vi "Actor Core.vi"(8 "error in":errorcluster, 11 "Splitter Settings UI in":refnum<class "Splitter Settings UI.lvclass">) -> (0 "error out":errorcluster, 3 "Actor out":refnum<class "Actor.lvclass">)   [LabVIEW 2020, in "Splitter Settings UI.lvlib" / "Splitter Settings UI.lvclass"]
doc: "The user interface for this panel.\n\n----\nPlease see the following web address for additional documentation and tutorial information:\nhttp://www.mooregoodideas.com/mgi-panel-manager/\n\nAuthor: Derek Trepanier\n\nCopyright (c) 2018, Moore Good Ideas, Inc.\n\nAll rights reserved.\n\nRedistribution and use in source and binary forms, with or without modification, are permitted provided that the following conditions are met:\n\n * Redistributions of source code must retain the above copyright notice, this list of conditions and the following disclaimer.\n * Redistributions in binary form must reproduce the above copyright notice, this list of conditions and the following disclaimer in the documentation and/or other materials provided with the distribution.\n * Neither the name of Moore Good Ideas, Inc. nor the names of its contributors may be used to endorse or promote products derived from this software without specific prior written permission.\n\nTHIS SOFTWARE IS PROVIDED BY THE COPYRIGHT HOLDERS AND CONTRIBUTORS \"AS IS\" AND ANY EXPRESS OR IMPLIED WARRANTIES, INCLUDING, BUT NOT LIMITED TO, THE IMPLIED WARRANTIES OF MERCHANTABILITY AND FITNESS FOR A PARTICULAR PURPOSE ARE DISCLAIMED. IN NO EVENT SHALL THE COPYRIGHT OWNER OR CONTRIBUTORS BE LIABLE FOR ANY DIRECT, INDIRECT, INCIDENTAL, SPECIAL, EXEMPLARY, OR CONSEQUENTIAL DAMAGES (INCLUDING, BUT NOT LIMITED TO, PROCUREMENT OF SUBSTITUTE GOODS OR SERVICES; LOSS OF USE, DATA, OR PROFITS; OR BUSINESS INTERRUPTION) HOWEVER CAUSED AND ON ANY THEORY OF LIABILITY, WHETHER IN CONTRACT, STRICT LIABILITY, OR TORT (INCLUDING NEGLIGENCE OR OTHERWISE) ARISING IN ANY WAY OUT OF THE USE OF THIS SOFTWARE, EVEN IF ADVISED OF THE POSSIBILITY OF SUCH DAMAGE."
uses:
  Splitter Settings UI.lvclass
  C:/Program Files (x86)/National Instruments/LabVIEW 2020/vi.lib/MGI/Panel Manager/Panel Actor/Panel Actor/Panel Actor.lvclass
  C:/Program Files (x86)/National Instruments/LabVIEW 2020/vi.lib/ActorFramework/Actor/Actor.lvclass
  <vilib>/ActorFramework/Actor/Actor.lvclass
  Typedefs/Splitter Style--Enum.ctl
  Splitter/Splitter.lvclass
  <vilib>/ActorFramework/Actor/Actor.lvclass/Actor.ctl
  <vilib>/ActorFramework/Message Enqueuer/Message Enqueuer.lvclass/Message Enqueuer.ctl
  Splitter Settings UI.lvclass/Splitter Settings UI.ctl
  Splitter Settings UI Messages/Set Cursor Busy State Msg/Set Cursor Busy State Msg.lvclass/Set Cursor Busy State Msg.ctl
  <vilib>/ActorFramework/Message Enqueuer/Init from Existing Queue.vi
  <vilib>/ActorFramework/Message Enqueuer/Enqueue.vi
  Pane Relief Main UI/Pane Relief Main UI Messages/Panel Object Settings Changed Msg/Panel Object Settings Changed Msg.lvclass
  C:/Program Files (x86)/National Instruments/LabVIEW 2020/vi.lib/ActorFramework/Message/Message.lvclass
  Splitter Settings UI Messages/Set Cursor Busy State Msg/Set Cursor Busy State Msg.lvclass
  <vilib>/ActorFramework/Message Priority Queue/Priority Enqueue.vi
  <vilib>/ActorFramework/Message Enqueuer/Message Enqueuer.lvclass
  <vilib>/MGI/Panel Manager/Panel Actor/Panel Actor/Panel Actor.lvclass
panel:
  in  "Label":string
  in  "Refresh Style Value":bool
  in  "Style":T1 items=["Modern", "Classic", "System", "NXG"]
  in  "Size":i32 min=0
  in  "Color":u32(colorbox)
  in  "Locked":bool
  in  "Sizing":u16(ring) items=["Sticks Top", "Sticks Bottom", "Proportional"]
  in  "Position":i32
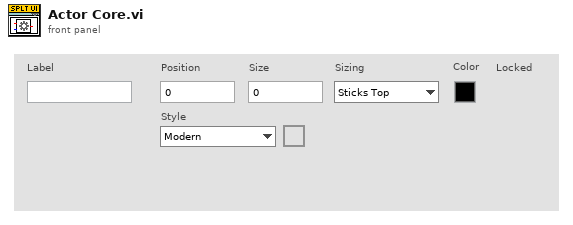
[diagram p1: front panel]
types:
  T1 = typedef "Splitter Style--Enum.ctl" = u16
  T2 = cluster{"Event Registration Refnum":refnum<event-registration>, "Pnl Actor":refnum<event-registration>}
  T3 = typedef "Splitter Sizing--Enum.ctl" = enum16{"Sticks Top/Left", "Sticks Bottom/Right", "Proportional"}
  T4 = typedef "Splitter Orientation--Enum.ctl" = enum16{"Vertical", "Horizontal"}
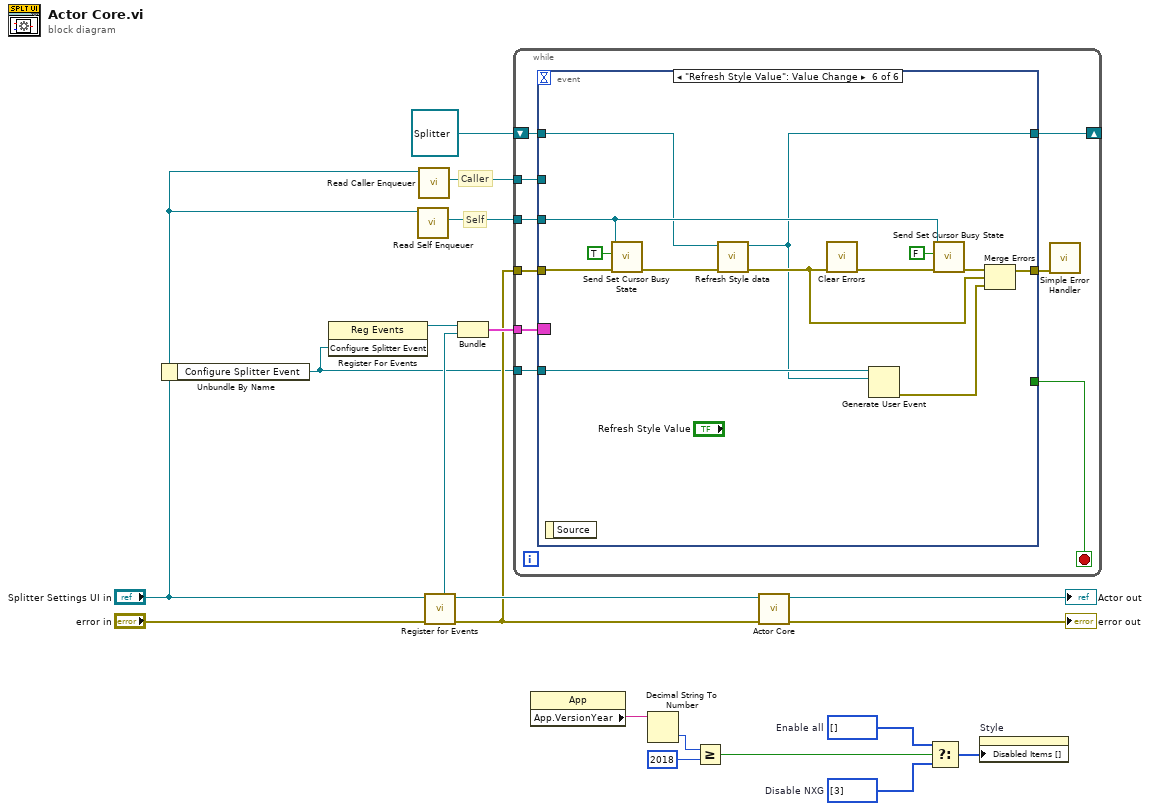
[diagram p0: block diagram]
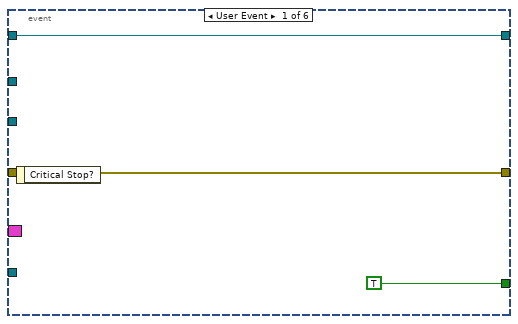
[diagram p2: hidden frame]
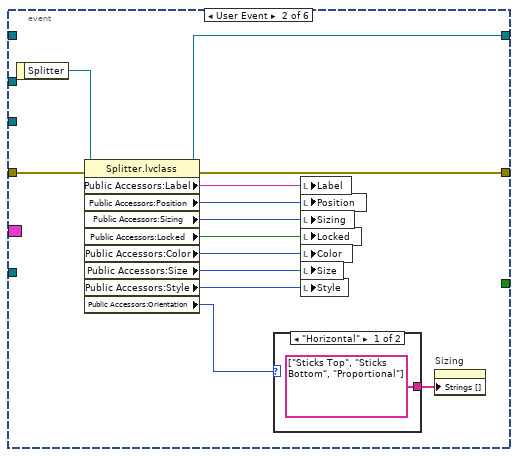
[diagram p3: hidden frame]
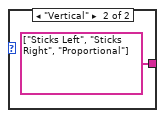
[diagram p4: hidden frame]
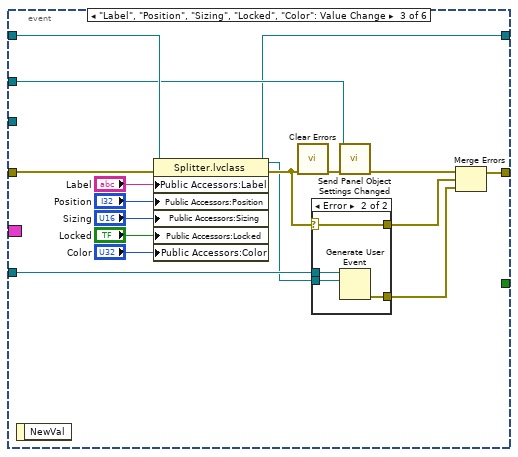
[diagram p5: hidden frame]
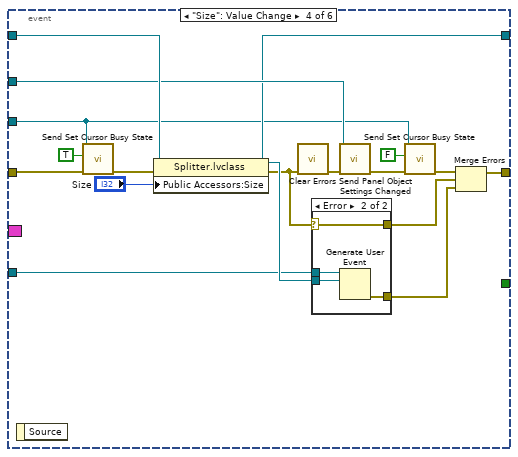
[diagram p7: hidden frame]
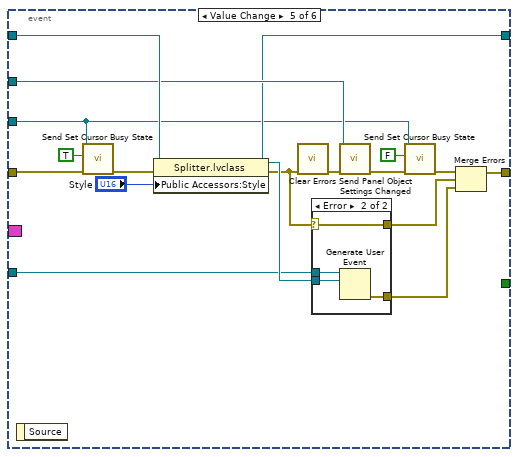
[diagram p9: hidden frame]
diagram:
  w3 = i32[] []  # Enable all
  w2 = i32[] [3]  # Disable NXG
  # "Self"
  # "Caller"
  n1 = Unbundle By Name("Splitter Settings UI in") -> ("Configure Splitter Event"=w10:refnum<user-event>)
  n2 = register-events(w10) -> (reference out=w16:refnum<event-registration>)  [unwired: 2 in, 1 out]
  n3 = call <vilib>:"Read Self Enqueuer.vi"("Actor"="Splitter Settings UI in") -> ("Self Enqueuer"=w9:refnum<class "Message Enqueuer.lvclass">)  [unwired: 10 in]
  n4 = call <vilib>:"Read Caller Enqueuer.vi"("Actor"="Splitter Settings UI in") -> ("Caller Enqueuer"=w11:refnum<class "Message Enqueuer.lvclass">)  [unwired: 10 in]
  n5 = call <vilib>:"Register for Events.vi"("Error In"="error in", "Panel Actor in"="Splitter Settings UI in") -> ("Error Out"=w12:errorcluster, "Panel Actor out"=w18:refnum<class "Splitter Settings UI.lvclass">, "Pnl Actor"=w15:refnum<event-registration>)  [unwired: 6 in, 1 out]
  n6 = Bundle("Event Registration Refnum"=w16, "Pnl Actor"=w15) -> (w14:T2)  [unwired: 1 in]
  n7 = while {
    tunnel: w14 -> [w29]
    shift-right: [w27] -> _
    shift-left: refnum<class "Splitter.lvclass"> refnum ("Splitter.lvclass") -> [w26]
    tunnel: w11 -> [w24]
    tunnel: w12 -> [w25]
    tunnel: w10 -> [w22]
    tunnel: w9 -> [w21]
    stop <- w28 stop-if-true
    n8 = event shown="[5] \"Refresh Style Value\": Value Change" {
      selector: w29 -> [_ _ _ _ _ _]
      dyn-events: _ -> [_ _ _ _ _ _]
      timeout: _ -> [_ _ _ _ _ _]
      tunnel: [TRUE _ _ _ _ _] -> w28
      tunnel: [w32 w38 w49 w78 w101 w113] -> w27
      tunnel: w26 -> [w32 _ w57 w85 w107 w114]
      tunnel: w25 -> [w31 w40 w58 w73 w96 w120]
      tunnel: [w31 w39 w53 w82 w105 w125] -> w23
      tunnel: w24 -> [_ _ w55 w81 w104 _]
      tunnel: w22 -> [_ _ w50 w76 w99 w122]
      tunnel: w21 -> [_ _ _ w71 w94 w118]
      event User Event {
        n9 = event-data() -> ()  [unwired: 1 in, 1 out]
      }
      event User Event {
        n10 = event-data() -> ("Splitter"=w37:refnum<class "Splitter.lvclass">)  [unwired: 1 in]
        n11 = property class="Splitter.lvclass"(reference=w37, error in=w40) -> (reference out=w38:refnum<class "Splitter.lvclass">, error out=w39:errorcluster, "Public Accessors:Label"=w45:string, "Public Accessors:Position"=w44:i32, "Public Accessors:Sizing"=w43:T3, "Public Accessors:Locked"=w42:bool, "Public Accessors:Color"=w41:u32, "Public Accessors:Size"=w36:i32, "Public Accessors:Style"=w33:T1, "Public Accessors:Orientation"=w35:T4)
        n12 = case shown="\"Horizontal\"" w35 {
          tunnel: [string[] ["Sticks Top", "Sticks Bottom", "Proportional"] ("Strings []") string[] ["Sticks Left", "Sticks Right", "Proportional"] ("Strings []")] -> w34
          frame "Horizontal" {
          }
          frame "Vertical" {
          }
        }
        n13 = local write "Label"(w45) -> ()
        n14 = local write "Position"(w44) -> ()
        n15 = local write "Sizing"(w43) -> ()
        n16 = local write "Locked"(w42) -> ()
        n17 = local write "Color"(w41) -> ()
        n18 = local write "Size"(w36) -> ()
        n19 = local write "Style"(w33) -> ()
        n20 = property on="Sizing" class="Ring (strict)"("Strings []"=w34) -> ()  [unwired: 2 in, 2 out]
      }
      event "Label", "Position", "Sizing", "Locked", "Color": Value Change {
        n21 = event-data() -> ()  [unwired: 1 in, 1 out]
        n22 = property class="Splitter.lvclass"(reference=w57, error in=w58, "Public Accessors:Label"="Label", "Public Accessors:Position"="Position", "Public Accessors:Sizing"="Sizing", "Public Accessors:Locked"="Locked", "Public Accessors:Color"="Color") -> (reference out=w49:refnum<class "Splitter.lvclass">, error out=w51:errorcluster)
        n23 = call <vilib>:"Clear Errors.vi"("error in (no error)"=w51) -> ("error out"=w56:errorcluster)  [unwired: 5 in, 1 out]
        n24 = case shown="Error" w51 {
          selector: w51 -> [w64 w68]
          tunnel: [w64 w68] -> w52
          tunnel: w50 -> [_ w67]
          tunnel: w49 -> [_ w66]
          tunnel: [_ w65] -> w48
          frame No Error {
          }
          frame Error {
            n25 = Generate User Event(user event=w67, event data cluster=w66) -> (error out=w65:errorcluster)  [unwired: 2 in, 1 out]
          }
        }
        n26 = call "Send Panel Object Settings Changed.vi"("error in (no error)"=w56, "Message Enqueuer"=w55) -> ("error out"=w54:errorcluster)  [unwired: 8 in, 1 out]
        n27 = Merge Errors(w54, w52, w48) -> (w53:errorcluster)
      }
      event "Size": Value Change {
        n28 = event-data() -> ()  [unwired: 1 in, 1 out]
        n29 = call "Send Set Cursor Busy State.vi"("error in (no error)"=w73, "Busy?"=TRUE, "Message Enqueuer"=w71) -> ("error out"=w74:errorcluster)  [unwired: 7 in, 1 out]
        n30 = property class="Splitter.lvclass"(reference=w85, error in=w74, "Public Accessors:Size"="Size") -> (reference out=w78:refnum<class "Splitter.lvclass">, error out=w77:errorcluster)
        n31 = call <vilib>:"Clear Errors.vi"("error in (no error)"=w77) -> ("error out"=w83:errorcluster)  [unwired: 5 in, 1 out]
        n32 = case shown="Error" w77 {
          selector: w77 -> [w86 w90]
          tunnel: [w86 w90] -> w80
          tunnel: w76 -> [_ w89]
          tunnel: w78 -> [_ w88]
          tunnel: [_ w87] -> w79
          frame No Error {
          }
          frame Error {
            n33 = Generate User Event(user event=w89, event data cluster=w88) -> (error out=w87:errorcluster)  [unwired: 2 in, 1 out]
          }
        }
        n34 = call "Send Panel Object Settings Changed.vi"("error in (no error)"=w83, "Message Enqueuer"=w81) -> ("error out"=w70:errorcluster)  [unwired: 8 in, 1 out]
        n35 = call "Send Set Cursor Busy State.vi"("error in (no error)"=w70, "Busy?"=FALSE, "Message Enqueuer"=w71) -> ("error out"=w69:errorcluster)  [unwired: 7 in, 1 out]
        n36 = Merge Errors(w69, w80, w79) -> (w82:errorcluster)
      }
      event Value Change {
        n37 = event-data() -> ()  [unwired: 1 in, 1 out]
        n38 = call "Send Set Cursor Busy State.vi"("error in (no error)"=w96, "Busy?"=TRUE, "Message Enqueuer"=w94) -> ("error out"=w97:errorcluster)  [unwired: 7 in, 1 out]
        n39 = property class="Splitter.lvclass"(reference=w107, error in=w97, "Public Accessors:Style"="Style") -> (reference out=w101:refnum<class "Splitter.lvclass">, error out=w100:errorcluster)
        n40 = call <vilib>:"Clear Errors.vi"("error in (no error)"=w100) -> ("error out"=w106:errorcluster)  [unwired: 5 in, 1 out]
        n41 = case shown="Error" w100 {
          selector: w100 -> [w108 w112]
          tunnel: [w108 w112] -> w103
          tunnel: w99 -> [_ w111]
          tunnel: w101 -> [_ w110]
          tunnel: [_ w109] -> w102
          frame No Error {
          }
          frame Error {
            n42 = Generate User Event(user event=w111, event data cluster=w110) -> (error out=w109:errorcluster)  [unwired: 2 in, 1 out]
          }
        }
        n43 = call "Send Panel Object Settings Changed.vi"("error in (no error)"=w106, "Message Enqueuer"=w104) -> ("error out"=w93:errorcluster)  [unwired: 8 in, 1 out]
        n44 = call "Send Set Cursor Busy State.vi"("error in (no error)"=w93, "Busy?"=FALSE, "Message Enqueuer"=w94) -> ("error out"=w92:errorcluster)  [unwired: 7 in, 1 out]
        n45 = Merge Errors(w92, w103, w102) -> (w105:errorcluster)
      }
      event "Refresh Style Value": Value Change {
        n46 = event-data() -> ()  [unwired: 1 in, 1 out]
        n47 = call "Send Set Cursor Busy State.vi"("error in (no error)"=w120, "Busy?"=TRUE, "Message Enqueuer"=w118) -> ("error out"=w115:errorcluster)  [unwired: 7 in, 1 out]
        n48 = call-dynamic "Refresh Style data.vi"("error in (no error)"=w115, "Splitter in"=w114) -> ("error out"=w124:errorcluster, "Splitter out"=w113:refnum<class "Splitter.lvclass">)  [unwired: 8 in]
        n49 = call <vilib>:"Clear Errors.vi"("error in (no error)"=w124) -> ("error out"=w117:errorcluster)  [unwired: 5 in, 1 out]
        n50 = Generate User Event(user event=w122, event data cluster=w113) -> (error out=w123:errorcluster)  [unwired: 2 in, 1 out]
        n51 = call "Send Set Cursor Busy State.vi"("error in (no error)"=w117, "Busy?"=FALSE, "Message Enqueuer"=w118) -> ("error out"=w116:errorcluster)  [unwired: 7 in, 1 out]
        n52 = Merge Errors(w116, w124, w123) -> (w125:errorcluster)
      }
    }
    n53 = call <vilib>:"Simple Error Handler.vi"("error in (no error)"=w23) -> ()  [unwired: 4 in, 5 out]
  }
  n54 = property class="App"() -> ("App.VersionYear"=w7:string)  [unwired: 2 in, 2 out]
  n55 = Decimal String To Number(string=w7) -> (number=w6:i32)  [unwired: 2 in, 1 out]
  n56 = Greater Or Equal?(x=w6, y=2018) -> (x >= y?=w4:bool)
  n57 = call-parent "Actor Core.vi"("error in"=w12, "Panel Actor in"=w18) -> ("error out"=→"error out":errorcluster, "Actor out"=→"Actor out":refnum<class "Actor.lvclass">)  [unwired: 8 in]
  n58 = Select(t=w3, s=w4, f=w2) -> (s? t:f=w1:i32[])
  n59 = property on="Style" class="Ring (strict)"("Disabled Items []"=w1) -> ()  [unwired: 2 in, 2 out]
